vi "Configure ARB.vi"(7 "Enable ARB (T:Enable)":bool=TRUE, 8 "error in (no error)":errorcluster, 10 "Runtime Scaling (70 percent)":dbl=70.0, 11 "VISA resource name":refnum<visa-resource-name>) -> (0 "error out":errorcluster, 3 "VISA resource name out":refnum<visa-resource-name>)   [LabVIEW 2012, in "Agilent PSG MXG Series.lvlib"]
doc: "Configures the arbitrary waveform generator.\n\n<B>Notes:</B>\n(1) This VI is valid only in E8267C, E8267D, N5162A, N5182A, N5172B, N5182B.\n\n(2) For E8267C, this VI is valid only when the instrument installs <B>Option 002</B> (Internal baseband generator) or <B>Option 602</B> (Digital bus baseband generator).\n\n(3) For E8267D, this VI is valid only when the instrument installs <B>Option 601</B> or <B>Option 602</B> (Internal baseband generator).\n\n(4) For N5162A and N5182A, this VI is valid only when the instrument installs <B>Option 651</B> or <B>Option 652</B> or <B>Option 654</B> (Internal baseband generator)."
uses:
  <instrlib>/Agilent PSG MXG Series/Agilent PSG MXG Series.lvlib
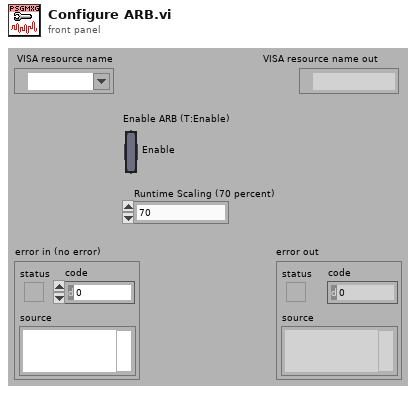
[diagram p1: front panel]
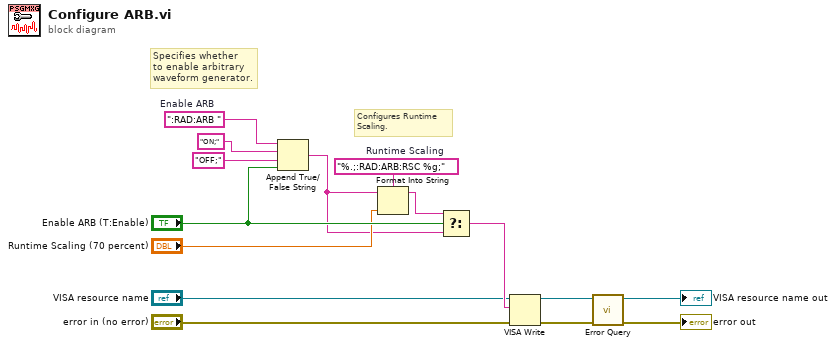
[diagram p0: block diagram]
diagram:
  w9 = "%.;:RAD:ARB:RSC %g;"  # Runtime Scaling
  w15 = ":RAD:ARB "  # Enable ARB
  # "Configures Runtime\nScaling."
  # "Specifies whether\nto enable arbitrary\nwaveform generator."
  n1 = Append True/False String(1:"Enable ARB (T:Enable)", 2:"OFF;" ("false string"), 3:"ON;" ("true string"), 4:w15) -> (0:w5:string)
  n2 = Format Into String(format string=w9, initial string=w5, "Runtime Scaling (70 percent)") -> (resulting string=w6:string)  [unwired: 1 in, 1 out]
  n3 = Select(t=w6, s="Enable ARB (T:Enable)", f=w5) -> (s? t:f=w10:string)
  n4 = VISA Write(VISA resource name="VISA resource name", write buffer=w10, error in (no error)="error in (no error)") -> (VISA resource name out=w12:refnum<visa-resource-name>, error out=w11:errorcluster)  [unwired: 1 out]
  n5 = call <instrlib>:"Error Query.vi"("error in (no error)"=w11, "VISA resource name"=w12) -> ("error out"=→"error out":errorcluster, "VISA resource name out"=→"VISA resource name out":refnum<visa-resource-name>)  [unwired: 8 out]
